vi "Check Level Limit.vi"(0 "Pin Names":string[](array[string]), 7 "Error from Limit":errorcluster[](array[cluster]), 11 "Error from Level":errorcluster[](array[cluster])) -> (4 "Error":string[](array[string]), 15 "error out":errorcluster)   [LabVIEW 2024, in "devicePowerSequencerCoreLogic.lvlib"]
uses:
  devicePowerSequencerCoreLogic.lvlib
  <vilib>/Utility/error.llb/Trim Whitespace One-Sided.vi
  <vilib>/Utility/error.llb/Clear Errors.vi
  Form Error Message.vi/4da3fa3f-d6a2-4c6b-9c9c-fc44bca91f7b.vi
  <vilib>/Utility/error.llb/Error Cluster From Error Code.vi
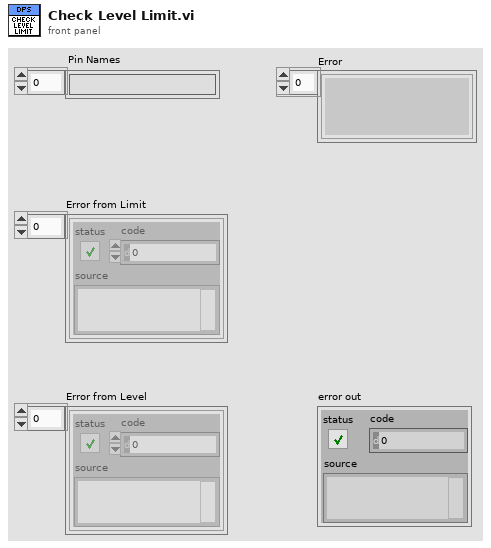
[diagram p1: front panel]
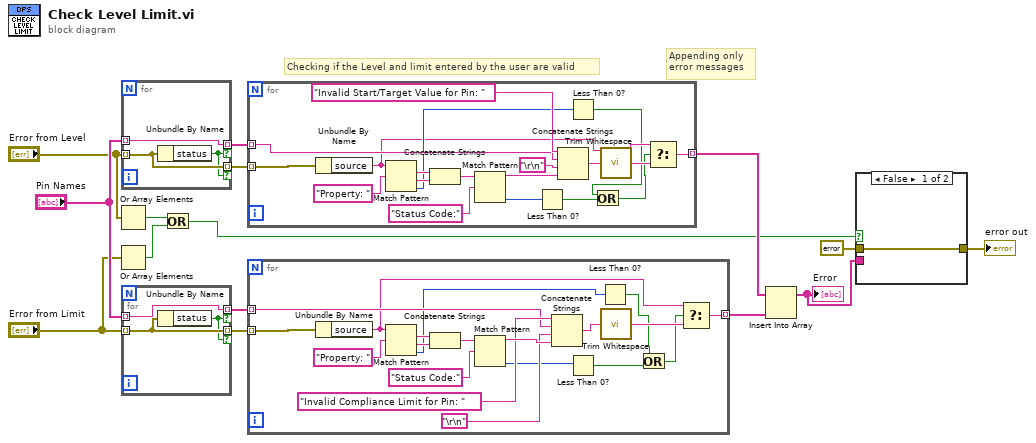
[diagram p0: block diagram]
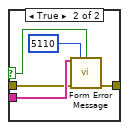
[diagram p2: hidden frame]
diagram:
  # "Checking if the Level and limit entered by the user are valid"
  # "Appending only\nerror messages"
  n1 = Or Array Elements(Boolean array="Error from Level") -> (logical OR=w8:bool)
  n2 = Or Array Elements(Boolean array="Error from Limit") -> (logical OR=w7:bool)
  n3 = for {
    tunnel: "Error from Level" -> [w18] mode=indexing
    tunnel: [w18] -> w15 mode=indexing if=w16
    tunnel: "Pin Names" -> [w17] mode=indexing
    tunnel: [w17] -> w13 mode=indexing if=w16
    n4 = Unbundle By Name(w18) -> ("status"=w16:bool)
  }
  n5 = for {
    tunnel: "Error from Limit" -> [w21] mode=indexing
    tunnel: [w21] -> w11 mode=indexing if=w19
    tunnel: "Pin Names" -> [w20] mode=indexing
    tunnel: [w20] -> w12 mode=indexing if=w19
    n6 = Unbundle By Name(w21) -> ("status"=w19:bool)
  }
  n7 = Or(x=w8, y=w7) -> (x .or. y?=w4:bool)
  n8 = for {
    tunnel: w15 -> [w40] mode=indexing
    tunnel: [w26] -> w10 mode=indexing
    tunnel: w13 -> [w31] mode=indexing
    n9 = Unbundle By Name(w40) -> ("source"=w28:string)
    n10 = Match Pattern(string=w28, regular expression="Property: ") -> (match substring=w37:string, after substring=w36:string, offset past match=w29:i32)  [unwired: 1 in, 1 out]
    n11 = Concatenate Strings(w37, w36) -> (w35:string)
    n12 = Match Pattern(string=w35, regular expression="Status Code:") -> (before substring=w34:string, offset past match=w25:i32)  [unwired: 1 in, 2 out]
    n13 = Less Than 0?(x=w25) -> (x < 0?=w24:bool)
    n14 = Concatenate Strings("Invalid Start/Target Value for Pin: " ("string"), w31, "\r\n", w34) -> (w32:string)
    n15 = Less Than 0?(x=w29) -> (x < 0?=w23:bool)
    n16 = Or(x=w23, y=w24) -> (x .or. y?=w22:bool)
    n17 = call <vilib>:"Trim Whitespace.vi"("string"=w32) -> ("trimmed string"=w27:string)  [unwired: 1 in]
    n18 = Select(t=w28, s=w22, f=w27) -> (s? t:f=w26:string)
  }
  n19 = for {
    tunnel: w11 -> [w59] mode=indexing
    tunnel: [w45] -> w9 mode=indexing
    tunnel: w12 -> [w50] mode=indexing
    n20 = Unbundle By Name(w59) -> ("source"=w47:string)
    n21 = Match Pattern(string=w47, regular expression="Property: ") -> (match substring=w56:string, after substring=w55:string, offset past match=w48:i32)  [unwired: 1 in, 1 out]
    n22 = Concatenate Strings(w56, w55) -> (w54:string)
    n23 = Match Pattern(string=w54, regular expression="Status Code:") -> (before substring=w53:string, offset past match=w44:i32)  [unwired: 1 in, 2 out]
    n24 = Concatenate Strings("Invalid Compliance Limit for Pin: " ("string"), w50, "\r\n", w53) -> (w51:string)
    n25 = Less Than 0?(x=w44) -> (x < 0?=w43:bool)
    n26 = Less Than 0?(x=w48) -> (x < 0?=w42:bool)
    n27 = call <vilib>:"Trim Whitespace.vi"("string"=w51) -> ("trimmed string"=w46:string)  [unwired: 1 in]
    n28 = Or(x=w42, y=w43) -> (x .or. y?=w41:bool)
    n29 = Select(t=w47, s=w41, f=w46) -> (s? t:f=w45:string)
  }
  n30 = Insert Into Array(array=w10, new element=w9) -> (w6:string[])  [unwired: 1 in]
  "Error" <- w6
  n31 = case shown="False" w4 {
    selector: w4 -> [_ w62]
    tunnel: w6 -> [_ w65]
    tunnel: [w60 w64] -> w5
    tunnel: errorcluster {"status"=FALSE, "code"=0, "source"=""} ("error in (no error)") -> [w60 w61]
    frame False {
    }
    frame True {
      n32 = call "Form Error Message.vi"("Error Message"=w65, "error code (0)"=5110, "Error?"=w62, "error in (no error)"=w61) -> ("error out"=w64:errorcluster)  [unwired: 11 in]
    }
  }
  "error out" <- w5
